vi "VCI Read CAN Status.vi"(8 "error in (no error)":errorcluster, 9 "CANIndex":u32, 10 "DevIndex":u32, 11 "DevType":u32) -> (0 "error out":errorcluster, 2 "function return":u32, 3 "pCANStatus":T1)   [LabVIEW 2012, in "ControlCAN.lvlib"]
doc: "unsigned int WINAPI VCI_ReadCANStatus(unsigned int DevType,unsigned int DevIndex,unsigned int CANIndex,PVCI_CAN_STATUS pCANStatus);"
uses:
  ControlCAN.lvlib
  Ginkgo_Driver.dll
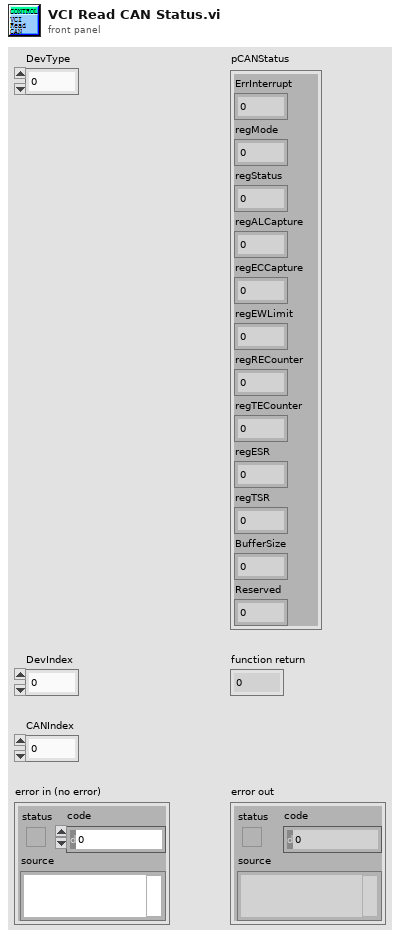
[diagram p1: front panel]
types:
  T1 = cluster{"ErrInterrupt":u8, "regMode":u8, "regStatus":u8, "regALCapture":u8, "regECCapture":u8, "regEWLimit":u8, "regRECounter":u8, "regTECounter":u8, "regESR":u32, "regTSR":u32, "BufferSize":u32, "Reserved":u32}
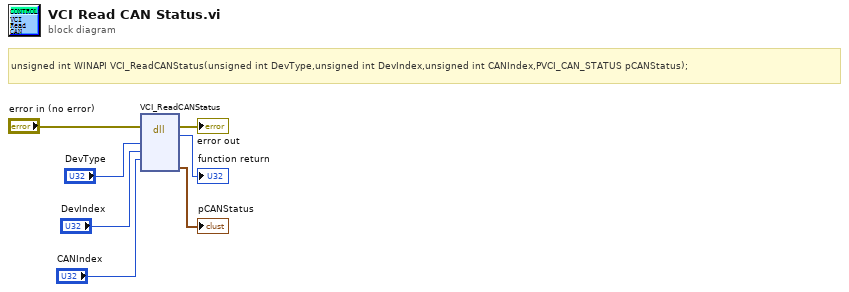
[diagram p0: block diagram]
diagram:
  # "unsigned int WINAPI VCI_ReadCANStatus(unsigned int DevType,unsigned int DevIndex,unsigned int CANIndex,PVCI_CAN_STATUS pCANStatus);"
  n1 = dll-call lib="E:/Project/vt_ginkgo/truck/Ginkgo Driver/vs2010/Ginkgo_USB-I2C_API_v2.0.3.0/lib/labview_32bit/ControlCAN/Ginkgo_Driver.*" fn="VCI_ReadCANStatus"(error in="error in (no error)", "DevType"="DevType", "DevIndex"="DevIndex", "CANIndex"="CANIndex") -> (error out=→"error out":errorcluster, →"function return":u32, "pCANStatus"=→"pCANStatus":T1)  [unwired: 6 in, 1 out]
